vi "Set All.vi"(8 "error in (no error)":errorcluster, 9 "Camera Settings":T1={"Exposure Time (ms)"=100.0, "Binning"=enum."2x2", "Scan Mode"=-1, "Frames to Acquire"=1000.0, "Pixel Correction"=FALSE, "Frames to Skip"=1, "File Path"=path "", "Duty cycle"=1.0, "ALEX"=FALSE, "Shutter Enable"=[], "fluidics trigger frame"=0, "Bit Depth"=16, "Image Width (px)"=0, "Image Height (px)"=0, "Horizontal Offset (px)"=0, "Vertical Offset (px)"=0} {"fluidics trigger frame" max=60000 step=1; "Exposure Time (ms)" min=1.0 max=10000.0 step=1.0}, 10 "Streaming?":bool, 11 "Synchronization Device in":refnum<class "Sync Device.lvclass">) -> (0 "error out":errorcluster, 3 "Synchronization Device out":refnum<class "Sync Device.lvclass">)   [LabVIEW 2023, in "Sync Device.lvlib" / "Sync Device.lvclass"]
uses:
  Sync Device.lvclass
  Resources/Type Defs/Camera Settings.ctl
  Sync Device.lvclass/Sync Device.ctl
  Resources/GLOBAL/GLOBAL Experiment Metadata.vi
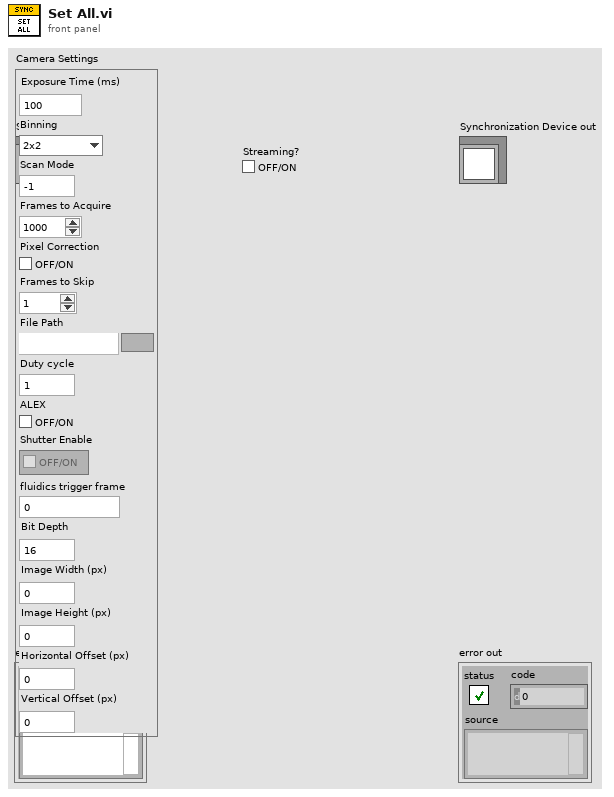
[diagram p1: front panel]
types:
  T1 = typedef "Camera Settings.ctl" = cluster{"Exposure Time (ms)":dbl, "Binning":enum16{"1x1", "2x2", "4x4"}, "Scan Mode":i32, "Frames to Acquire":dbl, "Pixel Correction":bool, "Frames to Skip":u32, "File Path":path, "Duty cycle":dbl, "ALEX":bool, "Shutter Enable":bool[], "fluidics trigger frame":u16, "Bit Depth":u16, "Image Width (px)":u16, "Image Height (px)":u16, "Horizontal Offset (px)":u16, "Vertical Offset (px)":u16}
  T2 = cluster{"Shutter Enable":bool[], "Duty Cycle":dbl, "Wavelengths":dbl[], "ALEX?":bool}
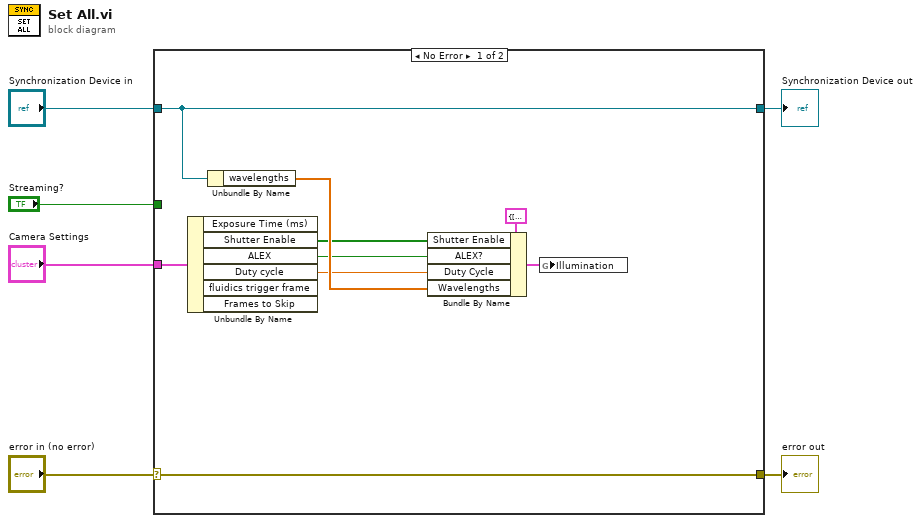
[diagram p0: block diagram]
diagram:
  n1 = case shown="No Error" "error in (no error)" {
    selector: "error in (no error)" -> [w7 w17]
    tunnel: [w7 w17] -> w5
    tunnel: [w15 w16] -> w3
    tunnel: "Synchronization Device in" -> [w15 w16]
    tunnel: "Streaming?" -> [_ _]
    tunnel: "Camera Settings" -> [w13 _]
    frame No Error {
      n2 = Unbundle By Name(w13) -> ("Shutter Enable"=w8:bool[], "ALEX"=w9:bool, "Duty cycle"=w12:dbl)  [unwired: 3 out]
      n3 = Unbundle By Name(w15) -> ("wavelengths"=w14:dbl[])
      n4 = Bundle By Name(cluster=T2 {"Shutter Enable"=[], "Duty Cycle"=0.0, "Wavelengths"=[], "ALEX?"=FALSE} ("Cluster"), "Shutter Enable"=w8, "ALEX?"=w9, "Duty Cycle"=w12, "Wavelengths"=w14) -> (w11:T2)
      n5 = global write "GLOBAL Experiment Metadata.vi" "Illumination"(w11) -> ()
    }
    frame Error {
    }
  }
  "error out" <- w5
  "Synchronization Device out" <- w3
